vi "Bulk Add DI Coil - Right Click.vi"(11 "Node Ptr":T1 format="%.0x") -> ()   [LabVIEW 2020, in "Modbus Master System Explorer.lvlib"]
uses:
  Modbus Master System Explorer.lvlib
  <vilib>/NI VeriStand/Custom Device API/Custom Device Item Ref.ctl
  Add DI Coil.vi
  <vilib>/NI VeriStand/Custom Device API/Custom Device API.lvlib
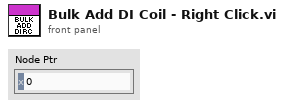
[diagram p1: front panel]
types:
  T1 = typedef "Custom Device API.lvlib/Custom Device Item Ref.ctl" = u64
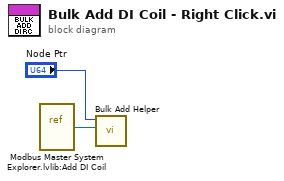
[diagram p0: block diagram]
diagram:
  n1 = vi-ref "Modbus Master System Explorer.lvlib:Add DI Coil.vi"() -> (w1:refnum<vi>)
  n2 = call "Bulk Add Helper.vi"("Add VI In"=w1, "Node Ptr"="Node Ptr") -> ()  [unwired: 10 in]
